vi "구획스크롤보이기(SubVI).vi"(10 "수직 스크롤 막대 보이기":T1(ring), 11 "Pane 입력":refnum<vi>) -> (0 "에러 출력":errorcluster)   [LabVIEW 2014]
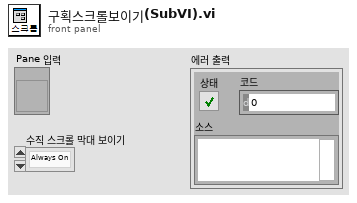
[diagram p1: front panel]
types:
  T1 = enum16{"Always On", "Always Off", "Off While Running"}
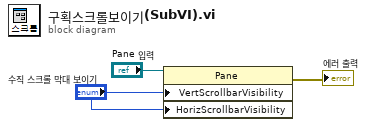
[diagram p0: block diagram]
diagram:
  n1 = property on="프로퍼티 노드" class="Pane"(reference="Pane 입력", "VertScrollbarVisibility"="수직 스크롤 막대 보이기", "HorizScrollbarVisibility"="수직 스크롤 막대 보이기") -> (error out=→"에러 출력":errorcluster)  [unwired: 1 in, 1 out]
